vi "HospitalInfo.vi"(11 "Notifier":refnum<notifier>) -> ()   [LabVIEW 2013, in "main.lvlib"]
uses:
  main.lvlib
  Controls/Enum Save Action Events.ctl
  Controls/Enum User Events.ctl
panel:
  in  "DepartmentStr":string caption="Afdeling"
  in  "AddressStr":string caption="Adresse"
  in  "HospitalStr":string caption="Hospital"
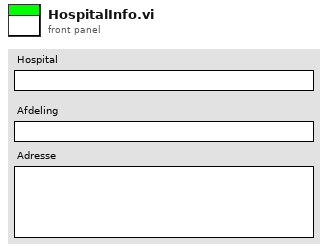
[diagram p1: front panel]
types:
  T1 = typedef "main.lvlib/Enum Save Action Events.ctl" = enum16{"LoadReportPath", "SaveReportPath", "Load Graph Path", "Save Graph Path", "LoadDataPath", "SaveDataPath", "Load Template Path", "Save Template Path", "Load PressureFactor", "Save PressureFactor", "Init", "Load Listbox", "Save Listbox", "LoadHospInfo", "SaveHospInfo", "Load DICOM Activation", "Save DICOM Activation", "LoadDICOMInfoWL", "SaveDICOMInfoWL", "LoadDICOMInfoPACS", "SaveDICOMInfoPACS", "Load ArmCalcMethod", "Save ArmCalcMethod", "LoadItemTags", "SaveItemTags", "LoadDICOMEncoding", "SaveDICOMEncoding", "LoadJournalType", "SaveJournalType", "LoadAcqFilterType", "SaveAcqFilterType", "Load Sequence", "Save Sequence", "Load Acquisition Mode", "Save Acquisition Mode", "Load General Settings", "Save General Settings", "Load Language", "Save Language", "Load Dicom Tags", "Save Dicom Tags", "Load BT Serial", "Save BT Serial", "Load BT License", "Save BT License"}
  T2 = cluster{"Name":string, "Address":string, "Department":string}
  T3 = typedef "main.lvlib/Enum User Events.ctl" = enum16{"User Event", "Init"}
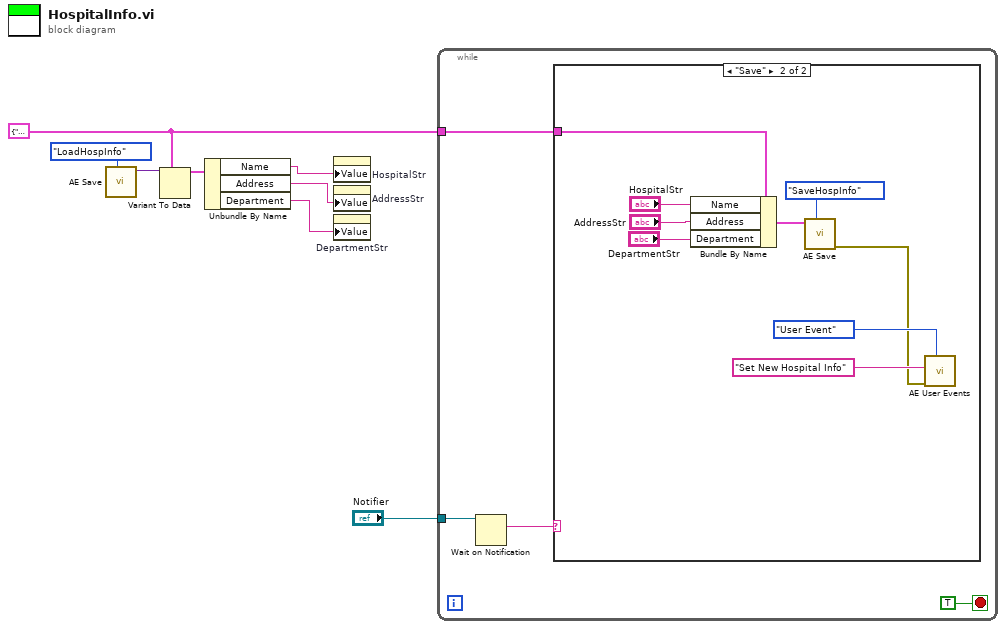
[diagram p0: block diagram]
diagram:
  w6 = T2 {"Name"="", "Address"="", "Department"=""} ("HospInfo")
  n1 = call "AE Save.vi"("Action"=Enum_Save_Action_Events."LoadHospInfo") -> ("Anything"=w7:variant)  [unwired: 8 in, 1 out]
  n2 = Variant To Data(type=w6, Variant=w7) -> (data=w5:T2)  [unwired: 1 in, 1 out]
  n3 = Unbundle By Name(w5) -> ("Name"=w4:string, "Address"=w3:string, "Department"=w2:string)
  n4 = property on="HospitalStr" class="Str"("Value"=w4) -> ()  [unwired: 2 in, 2 out]
  n5 = property on="AddressStr" class="Str"("Value"=w3) -> ()  [unwired: 2 in, 2 out]
  n6 = property on="DepartmentStr" class="Str"("Value"=w2) -> ()  [unwired: 2 in, 2 out]
  n7 = while {
    tunnel: w6 -> [w11]
    tunnel: "Notifier" -> [w9]
    stop <- TRUE stop-if-true
    n8 = Wait on Notification(notifier=w9) -> (notification=w12:string)  [unwired: 3 in, 3 out]
    n9 = case shown="\"Save\"" w12 {
      tunnel: w11 -> [_ w16]
      frame "Cancel", Default {
      }
      frame "Save" {
        n10 = Bundle By Name(cluster=w16, "Name"="HospitalStr", "Address"="AddressStr", "Department"="DepartmentStr") -> (w17:T2)
        n11 = call "AE Save.vi"("Variant In"=w17, "Action"=Enum_Save_Action_Events."SaveHospInfo") -> ("error out"=w13:errorcluster)  [unwired: 7 in, 1 out]
        n12 = call "AE User Events.vi"("Action"=Enum_User_Events."User Event", "error in (no error)"=w13, "User Event"="Set New Hospital Info") -> ()  [unwired: 7 in, 2 out]
      }
    }
  }
